vi "Trabalhando_arrays.vi"() -> ()   [LabVIEW 2020]
panel:
  in  "stop":bool
  out "Matriz 2D":dbl[][](array[numeric])
  in  "Escalar":dbl
  out "Matriz 1D (concatena 2 matrizes 1D + escalar intercalado)":dbl[](array[numeric])
  out "Matriz 1D (1D concatenada com 1D)":dbl[](array[numeric])
  in  "Matriz 1D":dbl[](array[numeric])
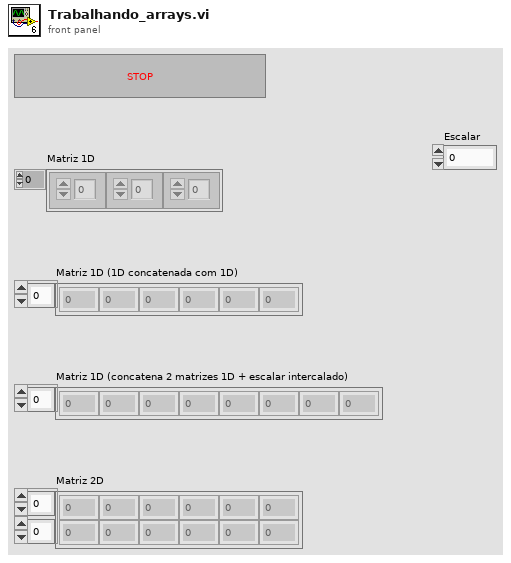
[diagram p1: front panel]
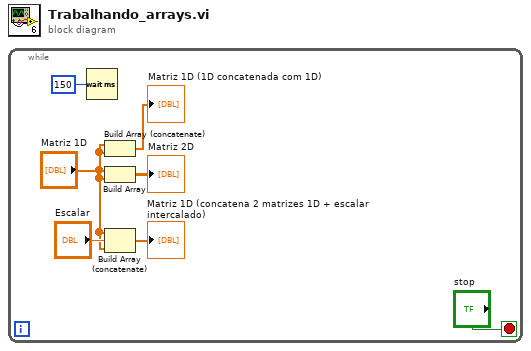
[diagram p0: block diagram]
diagram:
  n1 = while {
    stop <- "stop" stop-if-true
    n2 = Wait (ms)(milliseconds to wait=u32 150) -> ()  [unwired: 1 out]
    n3 = Build Array (concatenate)("Matriz 1D", "Matriz 1D") -> (→"Matriz 1D (1D concatenada com 1D)":dbl[])
    n4 = Build Array("Matriz 1D", "Matriz 1D") -> (→"Matriz 2D":dbl[][])
    n5 = Build Array (concatenate)("Matriz 1D", "Escalar", "Matriz 1D") -> (→"Matriz 1D (concatena 2 matrizes 1D + escalar intercalado)":dbl[])
  }
